vi "TPG261_ConvertData.vi"(11 "String in":string="2, 1.0100E+03,5, 0.0000E+00") -> (0 "DBL out":dbl[](array[numeric])=[2.0, 1.0, 5.0, 0.0], 1 "Integer Out":i32[](array[numeric])=[2, 1, 5, 0], 2 "Read Status":u16(ring)=1 items=["Read Failed", "Read Ok"], 3 "String out":string[](array[string])=["2", " 1.0100E+03", "5", " 0.0000E+00"], 4 "Array":string[](array[string])=["2", " 1,0100E+03", "5", " 0,0000E+00"])   [LabVIEW 2012]
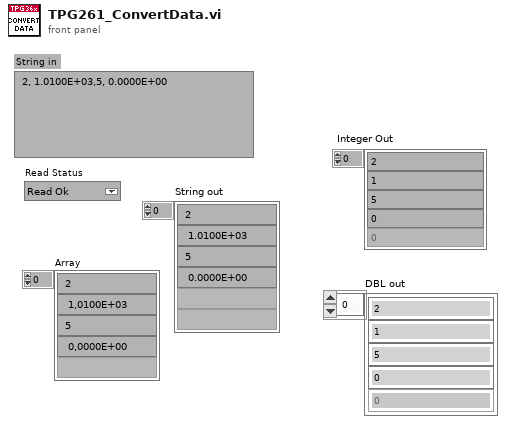
[diagram p1: front panel]
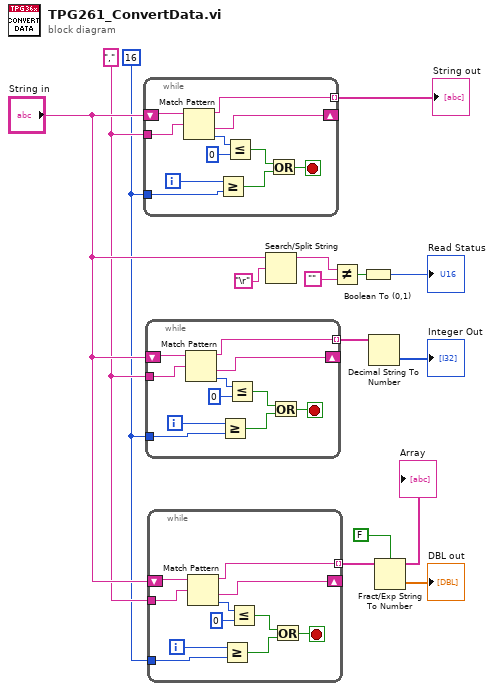
[diagram p0: block diagram]
diagram:
  w2 = 16 ("x")
  w4 = "," ("regular expression")
  n1 = while {
    shift-right: [w18] -> _
    shift-left: "String in" -> [w20]
    tunnel: [w19] -> w3 mode=indexing
    tunnel: w4 -> [w16]
    tunnel: w2 -> [w15]
    i -> [w21]
    stop <- w22 stop-if-true
    n2 = Match Pattern(string=w20, regular expression=w16) -> (before substring=w19:string, after substring=w18:string, offset past match=w17:i32)  [unwired: 1 in, 1 out]
    n3 = Greater Or Equal?(x=w21, y=w15) -> (x >= y?=w23:bool)
    n4 = Less Or Equal?(x=w17, y=0) -> (x <= y?=w24:bool)
    n5 = Or(x=w24, y=w23) -> (x .or. y?=w22:bool)
  }
  "String out" <- w3
  n6 = while {
    shift-right: [w29] -> _
    shift-left: "String in" -> [w31]
    tunnel: [w30] -> w12 mode=indexing
    tunnel: w4 -> [w27]
    tunnel: w2 -> [w26]
    i -> [w32]
    stop <- w33 stop-if-true
    n7 = Match Pattern(string=w31, regular expression=w27) -> (before substring=w30:string, after substring=w29:string, offset past match=w28:i32)  [unwired: 1 in, 1 out]
    n8 = Greater Or Equal?(x=w32, y=w26) -> (x >= y?=w34:bool)
    n9 = Less Or Equal?(x=w28, y=0) -> (x <= y?=w35:bool)
    n10 = Or(x=w35, y=w34) -> (x .or. y?=w33:bool)
  }
  n11 = while {
    shift-right: [w41] -> _
    shift-left: "String in" -> [w42]
    tunnel: [w37] -> w11 mode=indexing
    tunnel: w4 -> [w39]
    tunnel: w2 -> [w38]
    i -> [w43]
    stop <- w44 stop-if-true
    n12 = Match Pattern(string=w42, regular expression=w39) -> (before substring=w37:string, after substring=w41:string, offset past match=w40:i32)  [unwired: 1 in, 1 out]
    n13 = Greater Or Equal?(x=w43, y=w38) -> (x >= y?=w45:bool)
    n14 = Less Or Equal?(x=w40, y=0) -> (x <= y?=w46:bool)
    n15 = Or(x=w46, y=w45) -> (x .or. y?=w44:bool)
  }
  "Array" <- w11
  n16 = Search/Split String(string="String in", search string/char (-)="\r") -> (substring before match=w6:string)  [unwired: 1 in, 2 out]
  n17 = Not Equal?(x=w6, y="") -> (x != y?=w8:bool)
  n18 = Boolean To (0,1)(Boolean=w8) -> (0, 1=→"Read Status":i16)
  n19 = Decimal String To Number(string=w12) -> (number=→"Integer Out":i32[])  [unwired: 2 in, 1 out]
  n20 = Fract/Exp String To Number(use system decimal point (T)=FALSE, string=w11) -> (number=→"DBL out":dbl[])  [unwired: 2 in, 1 out]
